vi "SunplusDailyWIP1.vi"() -> ()   [LabVIEW 2012]
uses:
  <vilib>/addons/database/Auxilliary.llb/DB Tools Cursor Type.ctl
  <vilib>/Utility/NIReport.llb/NI_report.lvclass
  <vilib>/addons/database/Connection.llb/DB Tools Open Connec (Path).vi
  <vilib>/addons/database/Connection.llb/Conn Execute.vi
  <vilib>/addons/database/Recordset.llb/Rec Fetch Recordset Data (R).vi
  <vilib>/addons/database/Recordset.llb/Rec Destroy - Connection.vi
  <vilib>/addons/database/Recordset.llb/Rec Fetch Integer Data (R).vi
  <vilib>/Utility/NIReport.llb/Append Text Table to Report (wrap).vi
  <vilib>/addons/database/_DB Variant To Data/Database Variant To Data.xnode
  <vilib>/addons/database/NI_Database_API.lvlib
  <vilib>/Utility/NIReport.llb/Excel/NI_Excel.lvclass
panel:
  out "error out 2":errorcluster
  out "error out":errorcluster
  in  "template (empty)":path=path "O:/Monitor/Report/SunplusWIP.xls"
  out "array":string[][](array[string])
  out "appended array":string[](array[string])
  out "recordset data":variant[][](array[variant])
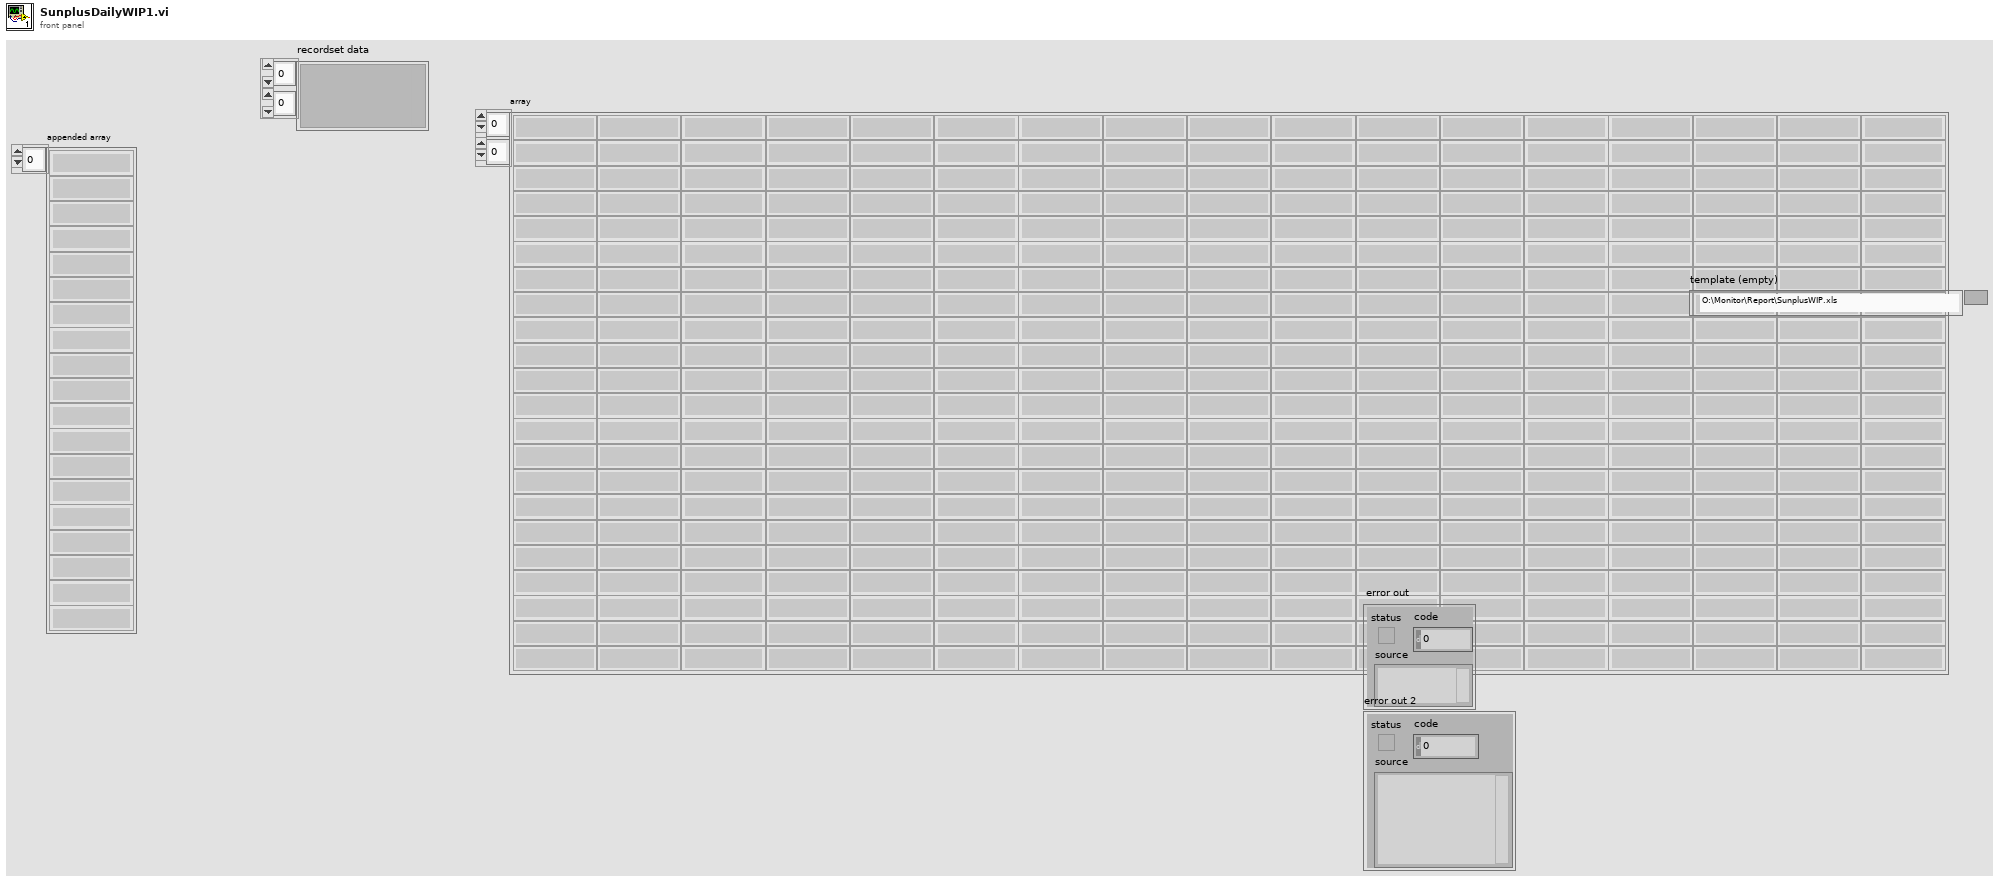
[diagram p1: front panel]
types:
  T1 = typedef "NI_Database_API.lvlib/DB Tools Cursor Type.ctl" = enum16{"forward-only", "keyset", "dynamic", "static"}
  T2 = typedef "NI_Database_API.lvlib/Conn ObjectReference.ctl" = refnum<k1>
  T3 = typedef "NI_Database_API.lvlib/Rec ObjectReference.ctl" = refnum<k1>
  T4 = enum16{"Standard Report", "HTML", "Word", "Excel"}
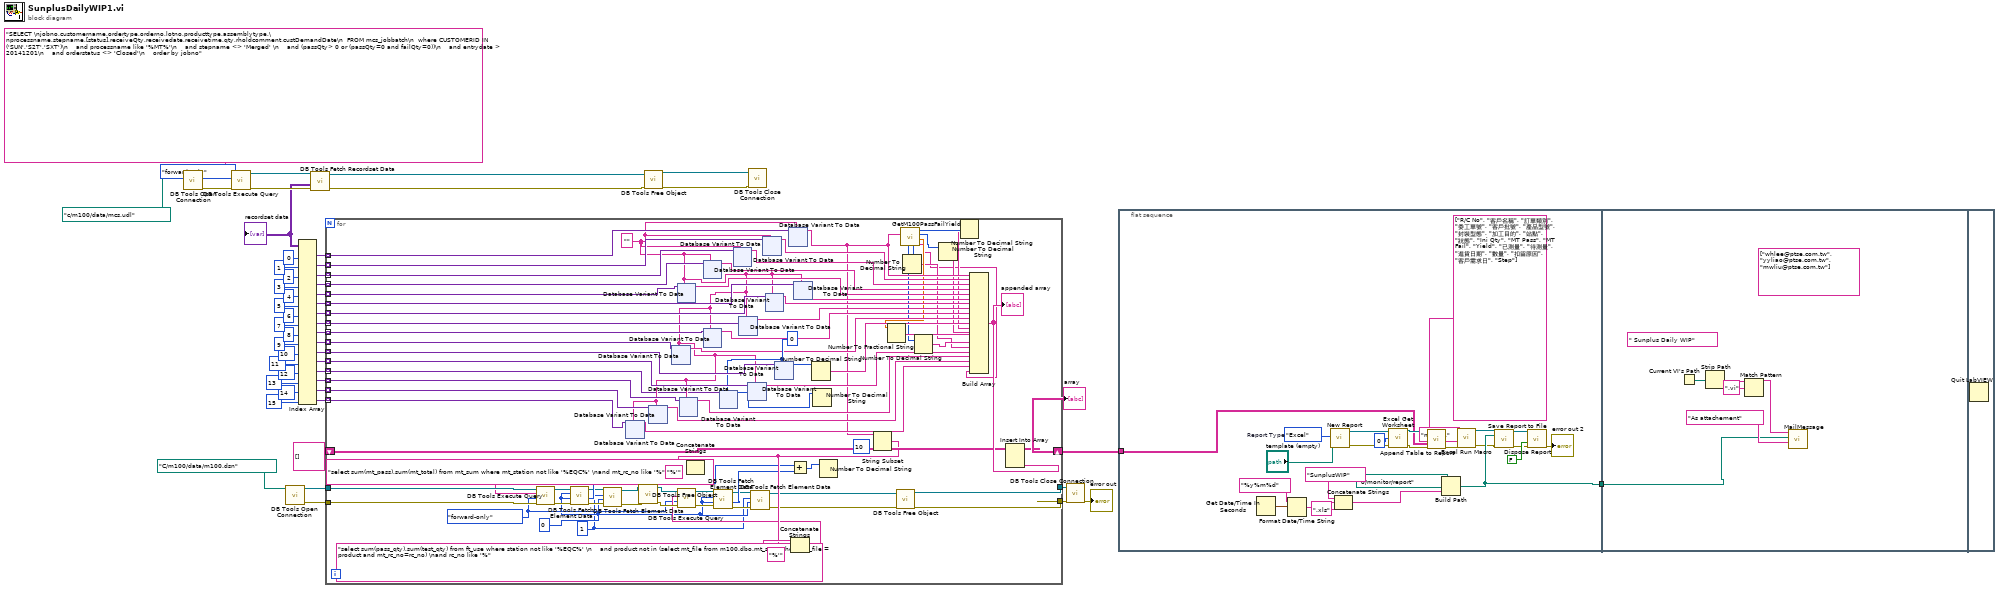
[diagram p0: block diagram]
diagram:
  n1 = call-poly <vilib>:"DB Tools Open Connection.vi"("connection information"=path "c:/m100/data/mcs.udl") -> ("error out"=w51:errorcluster, "connection reference"=w52:T2)  [unwired: 7 in]
  n2 = call-poly <vilib>:"DB Tools Execute Query.vi"("error in (no error)"=w51, "cursor type"=DB_Tools_Cursor_Type."forward-only", "SQL query"="SELECT \njobno,customername,ordertype,orderno,lotno,producttype,assemblytype,\nprocessname,stepname,[status],receiveQty,receivedate,receivetime,qty,rholdcomment,custDemandDate\n  FROM mcs_jobbatch\n  where CUSTOMERID IN ('SUN','S2T','SXT')\n    and processname like '%MT%'\n    and stepname <> 'Merged' \n    and (passQty> 0 or (passQty=0 and failQty=0))\n    and entrydate > 20141201\n    and orderstatus <> 'Closed'\n    order by jobno", "connection reference"=w52) -> ("error out"=w49:errorcluster, "recordset reference"=w50:T3)  [unwired: 4 in]
  n3 = call-poly <vilib>:"DB Tools Open Connection.vi"("connection information"=path "C:/m100/data/m100.dsn") -> ("error out"=w5:errorcluster, "connection reference"=w6:T2)  [unwired: 7 in]
  n4 = call-poly <vilib>:"DB Tools Fetch Recordset Data.vi"("error in (no error)"=w49, "recordset reference"=w50) -> ("error out"=w47:errorcluster, "recordset data"=w41:variant[][], "recordset reference out"=w48:T3)  [unwired: 3 in]
  "recordset data" <- w41
  n5 = Index Array(array=w41, index (col) #1=0 ("disabled index (col)"), index (col) #2=1 ("index (col)"), index (col) #3=2 ("index (col)"), index (col) #4=3 ("index (col)"), index (col) #5=4 ("index (col)"), index (col) #6=5 ("index (col)"), index (col) #7=6 ("index (col)"), index (col) #8=7 ("index (col)"), index (col) #9=8 ("index (col)"), index (col) #10=9 ("index (col)"), index (col) #11=10 ("index (col)"), index (col) #12=11 ("index (col)"), index (col) #13=12 ("index (col)"), index (col) #14=13 ("index (col)"), index (col) #15=14 ("index (col)"), index (col) #16=15 ("index (col)")) -> (element #1=w24:variant[], element #2=w23:variant[], element #3=w22:variant[], element #4=w21:variant[], element #5=w20:variant[], element #6=w19:variant[], element #7=w18:variant[], element #8=w17:variant[], element #9=w16:variant[], element #10=w15:variant[], element #11=w14:variant[], element #12=w13:variant[], element #13=w12:variant[], element #14=w11:variant[], element #15=w10:variant[], element #16=w8:variant[])  [unwired: 16 in]
  n6 = for {
    tunnel: w24 -> [w134] mode=indexing
    tunnel: w23 -> [w133] mode=indexing
    tunnel: w22 -> [w132] mode=indexing
    tunnel: w21 -> [w131] mode=indexing
    tunnel: w20 -> [w130] mode=indexing
    tunnel: w19 -> [w129] mode=indexing
    tunnel: w18 -> [w128] mode=indexing
    tunnel: w17 -> [w127] mode=indexing
    tunnel: w16 -> [w126] mode=indexing
    tunnel: w15 -> [w125] mode=indexing
    tunnel: w14 -> [w124] mode=indexing
    tunnel: w13 -> [w123] mode=indexing
    tunnel: w12 -> [w80] mode=indexing
    tunnel: w11 -> [w122] mode=indexing
    tunnel: w10 -> [w121] mode=indexing
    shift-right: [w107] -> w2
    shift-left: string[][] [] ("array") -> [w106]
    tunnel: w8 -> [w105] mode=indexing
    tunnel: w6 -> [w103]
    tunnel: w5 -> [w102]
    tunnel: [w90] -> w4
    tunnel: [w89] -> w3
    w66 = 1
    w84 = DB_Tools_Cursor_Type."forward-only" ("cursor type")
    w67 = 0
    w120 = 0
    w104 = ""
    n7 = xnode "Database Variant To Data"("database variant"=w105, "type"=w104) -> ("data"=w79:string)  [unwired: 1 in, 1 out]
    n8 = xnode "Database Variant To Data"("database variant"=w121, "type"=w104) -> ("data"=w78:string)  [unwired: 1 in, 1 out]
    n9 = xnode "Database Variant To Data"("database variant"=w125, "type"=w104) -> ("data"=w111:string)  [unwired: 1 in, 1 out]
    n10 = xnode "Database Variant To Data"("database variant"=w130, "type"=w104) -> ("data"=w116:string)  [unwired: 1 in, 1 out]
    n11 = xnode "Database Variant To Data"("database variant"=w122, "type"=w104) -> ("data"=w77:string)  [unwired: 1 in, 1 out]
    n12 = xnode "Database Variant To Data"("database variant"=w131, "type"=w104) -> ("data"=w117:string)  [unwired: 1 in, 1 out]
    n13 = xnode "Database Variant To Data"("database variant"=w126, "type"=w104) -> ("data"=w112:string)  [unwired: 1 in, 1 out]
    n14 = xnode "Database Variant To Data"("database variant"=w80, "type"=w120) -> ("data"=w109:i32)  [unwired: 1 in, 1 out]
    n15 = xnode "Database Variant To Data"("database variant"=w132, "type"=w104) -> ("data"=w118:string)  [unwired: 1 in, 1 out]
    n16 = xnode "Database Variant To Data"("database variant"=w127, "type"=w104) -> ("data"=w113:string)  [unwired: 1 in, 1 out]
    n17 = xnode "Database Variant To Data"("database variant"=w123, "type"=w104) -> ("data"=w76:string)  [unwired: 1 in, 1 out]
    n18 = xnode "Database Variant To Data"("database variant"=w133, "type"=w104) -> ("data"=w119:string)  [unwired: 1 in, 1 out]
    n19 = xnode "Database Variant To Data"("database variant"=w128, "type"=w104) -> ("data"=w114:string)  [unwired: 1 in, 1 out]
    n20 = xnode "Database Variant To Data"("database variant"=w124, "type"=w120) -> ("data"=w110:i32)  [unwired: 1 in, 1 out]
    n21 = xnode "Database Variant To Data"("database variant"=w134, "type"=w104) -> ("data"=w65:string)  [unwired: 1 in, 1 out]
    n22 = xnode "Database Variant To Data"("database variant"=w129, "type"=w104) -> ("data"=w115:string)  [unwired: 1 in, 1 out]
    n23 = Number To Decimal String(number=w110) -> (decimal integer string=w96:string)  [unwired: 1 in]
    n24 = Number To Decimal String(number=w109) -> ()  [unwired: 1 in, 1 out]
    n25 = String Subset(string=w65, length (rest)=10 ("length (rest)")) -> (substring=w87:string)  [unwired: 1 in]
    n26 = Concatenate Strings("select sum(mt_pass),sum(mt_total) from mt_sum where mt_station not like '%EQC%' \nand mt_rc_no like '%" ("SQL query"), w87, "%'" ("string")) -> (w97:string)
    n27 = call-poly <vilib>:"DB Tools Execute Query.vi"("error in (no error)"=w102, "cursor type"=w84, "SQL query"=w97, "connection reference"=w103) -> ("error out"=w100:errorcluster, "recordset reference"=w101:T3)  [unwired: 4 in]
    n28 = call-poly <vilib>:"DB Tools Fetch Element Data.vi"("error in (no error)"=w100, "type"=w67, "column index"=w67, "recordset reference"=w101) -> ("error out"=w73:errorcluster, "data"=w82:i32, "recordset reference out"=w75:T3)  [unwired: 3 in]
    n29 = call-poly <vilib>:"DB Tools Fetch Element Data.vi"("error in (no error)"=w73, "type"=w67, "column index"=w66, "recordset reference"=w75) -> ("error out"=w72:errorcluster, "recordset reference out"=w74:T3)  [unwired: 3 in, 1 out]
    n30 = call-poly <vilib>:"DB Tools Free Object.vi"("error in (no error)"=w72, "recordset reference"=w74) -> ("error out"=w93:errorcluster, "connection reference"=w94:T2)  [unwired: 8 in]
    n31 = Concatenate Strings("select sum(pass_qty),sum(test_qty) from ft_use where station not like '%EQC%' \n    and product not in (select mt_file from m100.dbo.mt_sum where mt_file = product and mt_rc_no=rc_no) \nand rc_no like '%" ("SQL query"), w87, "%'" ("string")) -> (w85:string)
    n32 = call-poly <vilib>:"DB Tools Execute Query.vi"("error in (no error)"=w93, "cursor type"=w84, "SQL query"=w85, "connection reference"=w94) -> ("error out"=w91:errorcluster, "recordset reference"=w92:T3)  [unwired: 4 in]
    n33 = call-poly <vilib>:"DB Tools Fetch Element Data.vi"("error in (no error)"=w91, "type"=w67, "column index"=w67, "recordset reference"=w92) -> ("error out"=w69:errorcluster, "data"=w81:i32, "recordset reference out"=w71:T3)  [unwired: 3 in]
    n34 = call-poly <vilib>:"DB Tools Fetch Element Data.vi"("error in (no error)"=w69, "type"=w67, "column index"=w66, "recordset reference"=w71) -> ("error out"=w68:errorcluster, "recordset reference out"=w70:T3)  [unwired: 3 in, 1 out]
    n35 = Add(x=w82, y=w81) -> (x+y=w83:i32)
    n36 = Number To Decimal String(number=w83) -> ()  [unwired: 1 in, 1 out]
    n37 = call-poly <vilib>:"DB Tools Free Object.vi"("error in (no error)"=w68, "recordset reference"=w70) -> ("error out"=w89:errorcluster, "connection reference"=w90:T2)  [unwired: 8 in]
    n38 = call "GetM100PassFailYield.vi"("RCNO"=w65) -> ("Step"=w54:string, "Yield"=w60:dbl, "Fail"=w62:i32, "Pass"=w64:i32, "待測"=w58:i32, "已測"=w57:i32)  [unwired: 5 in]
    n39 = Number To Fractional String(number=w60) -> (F-format string=w59:string)  [unwired: 3 in]
    n40 = Number To Decimal String(number=w58) -> (decimal integer string=w55:string)  [unwired: 1 in]
    n41 = Number To Decimal String(number=w57) -> (decimal integer string=w56:string)  [unwired: 1 in]
    n42 = Number To Decimal String(number=w62) -> (decimal integer string=w61:string)  [unwired: 1 in]
    n43 = Number To Decimal String(number=w64) -> (decimal integer string=w63:string)  [unwired: 1 in]
    n44 = Build Array(w65, w119, w118, w117, w116, w115, w114, w113, w112, w111, w96, w63, w61, w59, w56, w55, w76, w77, w78, w79, w54) -> (w108:string[])
    "appended array" <- w108
    n45 = Insert Into Array(array=w106, new element=w108) -> (w107:string[][])  [unwired: 2 in]
  }
  "array" <- w2
  n46 = call-poly <vilib>:"DB Tools Free Object.vi"("error in (no error)"=w47, "recordset reference"=w48) -> ("error out"=w45:errorcluster, "connection reference"=w46:T2)  [unwired: 8 in]
  n47 = call <vilib>:"DB Tools Close Connection.vi"("error in (no error)"=w45, "connection reference"=w46) -> ()  [unwired: 5 in, 1 out]
  n48 = call <vilib>:"DB Tools Close Connection.vi"("error in (no error)"=w3, "connection reference"=w4) -> ("error out"=→"error out":errorcluster)  [unwired: 5 in]
  n49 = flat-sequence {
    tunnel: w2 -> [w654]
    tunnel: [w653] -> w53
    tunnel: w53 -> [w673]
    frame #0 {
      w672 = T4."Excel"  # Report Type
      n50 = Get Date/Time In Seconds() -> (seconds since 1Jan1904=w659:timestamp)
      n51 = Format Date/Time String(time format string (%c)="%y%m%d", seconds (now)=w659) -> (date/time string=w657:string)  [unwired: 1 in]
      n52 = call <vilib>:"New Report.vi"("report type"=w672, "template (empty)"="template (empty)") -> ("report out"=w671:refnum<class "NI_report.lvclass">, "error out"=w670:errorcluster)  [unwired: 12 in]
      n53 = Concatenate Strings("SunplusWIP" ("string"), w657, ".xls" ("string")) -> (w660:string)
      n54 = call <vilib>:"Excel Get Worksheet.vi"("report in"=w671, "worksheet index (0)"=0, "error in (no error)"=w670) -> ("report out"=w667:refnum<class "NI_report.lvclass">, "error out"=w666:errorcluster)  [unwired: 11 in]
      n55 = call-poly <vilib>:"Append Table to Report.vi"("report in"=w667, "column headers"=string[] ["R/C No", "客戶名稱", "訂單類別", "委工單號", "客戶批號", "產品型號", "封裝型態", "加工目的", "站點", "狀態", "Ini Qty", "MT Pass", "MT Fail", "Yield", "已測量", "待測量", "進貨日期", "數量", "扣留原因", "客戶需求日", "Step"], "text data"=w654, "error in (no error)"=w666) -> ("report out"=w649:refnum<class "NI_report.lvclass">, "error out"=w652:errorcluster)  [unwired: 8 in, 2 out]
      n56 = Build Path(base path=path "o:/monitor/report", name or relative path=w660) -> (appended path=w653:path)
      n57 = call <vilib>:"Excel Run Macro.vi"("report in"=w649, "macro name"="macro1", "error in (no error)"=w652) -> ("report out"=w651:refnum<class "NI_report.lvclass">, "error out"=w650:errorcluster)  [unwired: 10 in, 1 out]
      n58 = call-dynamic "Save Report to File.vi"("report in"=w651, "report file path"=w653, "error in (no error)"=w650) -> ("report out"=w664:refnum<class "NI_report.lvclass">, "error out"=w663:errorcluster)  [unwired: 11 in]
      n59 = call-dynamic "Dispose Report.vi"("report in"=w664, "save changes? (F)"=FALSE, "error in (no error)"=w663) -> ("error out"=→"error out 2":errorcluster)  [unwired: 12 in]
    }
    frame #1 {
      (unwired) string[] ["whlee@ptse.com.tw", "yyliao@ptse.com.tw", "mwliu@ptse.com.tw"] ("recipients")
      (unwired) " Sunplus Daily WIP" ("subject ([No Subject])")
      n60 = Current VI's Path() -> (path=w678:path)
      n61 = Strip Path(path=w678) -> (name=w677:string)  [unwired: 1 out]
      n62 = Match Pattern(string=w677, regular expression=".vi") -> (before substring=w675:string)  [unwired: 1 in, 3 out]
      n63 = call "MailMessage.vi"("message"="As attachement", "file path"=w673, "program"=w675) -> ()  [unwired: 9 in]
    }
    frame #2 {
      n64 = Quit LabVIEW() -> ()  [unwired: 1 in]
    }
  }
